vi "MeasureAtFreq.vi"(8 "error in (no error)":errorcluster, 11 "NetA_AgNA in":refnum<class "NetA_AgNA.lvclass">) -> (0 "error out":errorcluster, 3 "NetA_AgNA out":refnum<class "NetA_AgNA.lvclass">)   [LabVIEW 2014, in "NetA_AgNA.lvclass"]
uses:
  NetA_AgNA.lvclass
panel:
  # "NOTE: This is just a placeholder for the Dynamic Dispatch method\nof Instruments class. It is not implemented here. Just an empty shell."
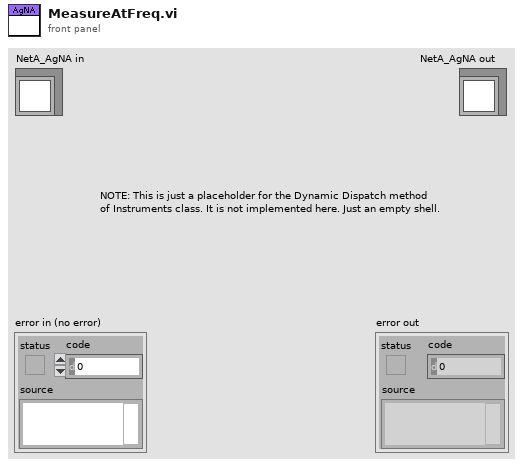
[diagram p1: front panel]
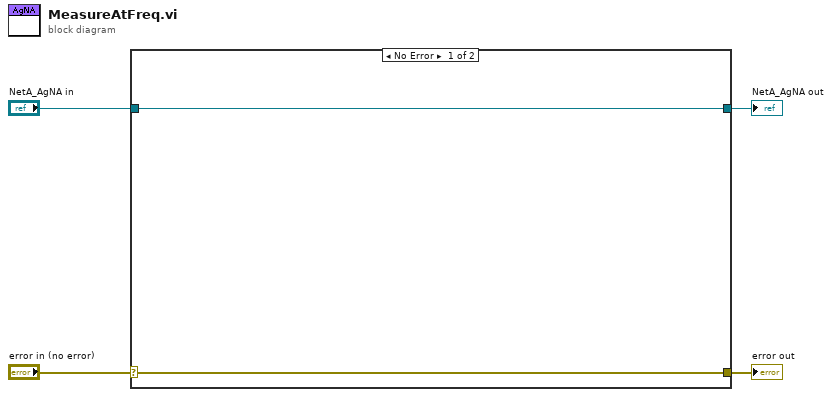
[diagram p0: block diagram]
diagram:
  n1 = case shown="No Error" "error in (no error)" {
    selector: "error in (no error)" -> [w5 w8]
    tunnel: [w5 w8] -> w3
    tunnel: [w6 w7] -> w1
    tunnel: "NetA_AgNA in" -> [w6 w7]
    frame No Error {
    }
    frame Error {
    }
  }
  "error out" <- w3
  "NetA_AgNA out" <- w1
